vi "SetRF.vi"(0 "reference in":refnum<class "niMmWave_Reciever.lvclass">, 5 "Port":string(combo), 7 "Frequency":dbl format="%#_6pHz", 9 "Gain":dbl format="%#_6fdb", 11 "error in (no error)":errorcluster) -> (4 "reference out":refnum<class "niMmWave_Reciever.lvclass">, 15 "error out":errorcluster)   [LabVIEW 2019, in "niMmWave_Reciever.lvclass"]
doc: "Set RF configuration for port:\nGain and frequency"
uses:
  niMmWave_Reciever.lvclass
  mmWave HW Control/LO sources.ctl
  mmWave HW Control/mmWave HW Control.lvlib
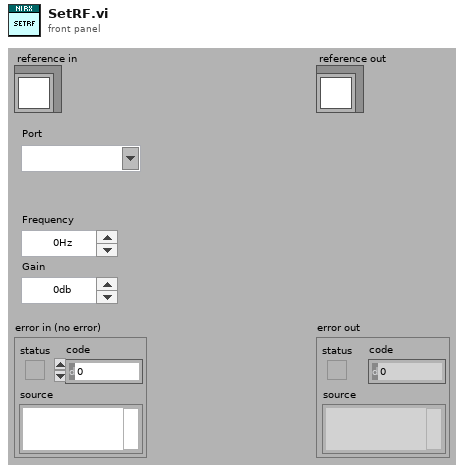
[diagram p1: front panel]
types:
  T1 = typedef "niMmWave_Reciever.lvclass/ObjectAttributesRef.ctl" = refnum<data-value>
  T2 = typedef "niMmWave_Reciever.lvclass/ObjectAttributes.ctl" = cluster{"session":T3[], "HW.RX devices":T17, "RF config":T18, "RX trigger options":T19, "RX samples":i32, "RX Fs":dbl}
  T3 = typedef "Session.ctl" = cluster{"3620 session":refnum<queue>, "tx baseband session":T4, "rx baseband session":T12, "tx gain (dB)":dbl, "rx gain (dB)":dbl, "hardware configuration":T13, "gain ranging":T15[], "pxi trigger bus information":T16}
  T4 = typedef "Tx Baseband Session.ctl" = cluster{"3610 session":T5, "7902 reference":T11}
  T5 = typedef "ni3610_and_ni3630_Driver_Lib.lvlib/Main Settings.ctl" = cluster{"VISA resource name":refnum<visa-resource-name>, "Address Space":T6, "window_offset":u32, "register_addresses":T7, "required_MM_fpga_version":cluster{"signature":u32, "hardware":u32, "current revision":u32, "oldest revision":u32}, "CPLD Oldest Compat Version ":cluster{"hardware":u32, "CPLD firmware":u32}, "MM_FPGA_image_location":string, "is_init":bool, "card_type":T8, "DacLmkConfigFileName":string, "AdcLmkConfigFileName":string, "AdcConfigFileName":string, "DacConfigFileName_RevA":string, "DacConfigFileName_RevB":string, "Mulde hardware revision":u8, "bypass DAC PLL\n":bool, "IQ Card Revision":T9, "board capability":T10}
  T6 = typedef "VISA Register Access Address Space.ctl" = u16
  T7 = typedef "ni3610_and_ni3630_Driver_Lib.lvlib/Register Adresses.ctl" = cluster{"MM based Registers":cluster{"Revision":u32, "OldestCompatRev":u32, "signature":u32, "scratch":u32, "LedControl":u32, "BoardHwRev":u32, "BoardControl":u32, "ThermalStatus":u32, "BasebandStatus":u32, "BasebandControl":u32, "BasebandAuxSetup":u32, "BasebandAuxStatus":u32, "LmkSyncOutSetup":u32, " AdcSyncOutSetup":u32, " InjSyncOutSetup":u32, " PxiTrig0OutSetup":u32, " PxiTrig1OutSetup":u32, " PxiTrig2OutSetup":u32, " PxiTrig3OutSetup":u32, " PxiTrig4OutSetup":u32, " PxiTrig5OutSetup":u32, " PxiTrig6OutSetup":u32, " PxiTrig7OutSetup":u32}, "CPLD based Registers":cluster{"SlaveSignature":u32, "SlaveRevision":u32, "SlaveOldestCompatRev":u32, "SlaveScratch":u32, "SlaveSetup":u32, "SlaveStatus":u32, "IDacReg_offset":u32, "LMKRegGrp0_offset":u32, "QDacReg_offset":u32, "BrdTempSensorVal":u32, "TempSensorPowerDown":u32, "GPIOReg_offset":u32, "IAdcReg_offset":u32, "QAdcReg_offset":u32, "LMKRegGrp1_offset":u32, "QadcTempSensorVal":u32, "IadcTempSensorVal":u32, "RevisionReg":u32, "VcxoReg":u32, "CpldStatusReg":u32, "PowerReg":u32, "VBiasEnReg":u32, "ExtRefOeReg":u32, "QdacCtrlReg":u32, "QdacStatusReg":u32, "IdacCtrlReg":u32, "IdacStatusReg":u32, "QdacJtagIn":u32, "QdacJtagOut":u32, "IdacJtagIn":u32, "IdacJtagOut":u32, "IqDcSetupReg":u32, "QadcStatusReg":u32, "IadcStatusReg":u32, "BrdSetupReg":u32, "IqDcRevisionReg":u32, "PllStatusReg":u32, "EndpointScratchReg":u32, "AdcSyncCfgReg":u32, "IqCardOpampReg":u32}, "CPLD Register Offset":u32, "MM  Register Offset":u32, " PxiTrig0OutSetup":u32}
  T8 = typedef "ni3610_and_ni3630_Driver_Lib.lvlib/Base Card Type.ctl" = enum16{"unspecified", "ADC", "DAC"}
  T9 = typedef "ni3610_and_ni3630_Driver_Lib.lvlib/IQ Card Revision.ctl" = enum16{"RevA", "RevB", "RevC", "RevD"}
  T10 = typedef "ni3610_and_ni3630_Driver_Lib.lvlib/Board Capability.ctl" = cluster{"baseband sync":enum16{"no baseband sync", "baseband sync"}}
  T11 = typedef "Blank FPGA Reference.ctl" = refnum<k20>
  T12 = typedef "Rx Baseband Session.ctl" = cluster{"3630 session":T5, "7902 reference":T11}
  T13 = typedef "Hardware Configuration.ctl" = cluster{"direction":T14, "baseband only":bool}
  T14 = typedef "Direction.ctl" = enum16{"Transceiver", "Receiver", "Transmitter"}
  T15 = typedef "Gain Ranging.ctl" = cluster{"gain ranging active scope":string, "gain ranging stream session":refnum<k20>}
  T16 = typedef "PXI Trigger Bus Info.ctl" = cluster{"chassis resource name":refnum<visa-resource-name>, "7902R (TX)":i16, "3610 (TX)":i16, "3620 (IF)":i16, "3630 (RX)":i16, "7902R (RX)":i16}
  T17 = typedef "mmWave HW Control.lvlib/HW RX resources cluster.ctl" = cluster{"HW.IF":tag, "HW.ADC":refnum<visa-resource-name>, "HW.RX FPGA":tag}
  T18 = typedef "mmWave HW Control.lvlib/HW RX RF config cluster.ctl" = cluster{"Gain":dbl, "Frequency":dbl, "mmWave adapter":string}
  T19 = typedef "TX trigger config.ctl" = cluster{"delay":dbl, "trig source":T20, "PXI src":i32, "export":T21, "PXI dest":i32}
  T20 = typedef "FPGA Utility.lvlib/FPGA driver trigger source.ctl" = enum16{"Use Tclk", "PXI_Trig", "Aurora RX trig"}
  T21 = typedef "FPGA Utility.lvlib/FPGA driver trigger destination.ctl" = enum16{"None", "Source trig", "Synced trig", "Delayed sync"}
  T22 = typedef "mmWave HW Control.lvlib/LO sources.ctl" = cluster{"RX/LO1 src":string, "TX/LO1 src":string, "LO2 src":string}
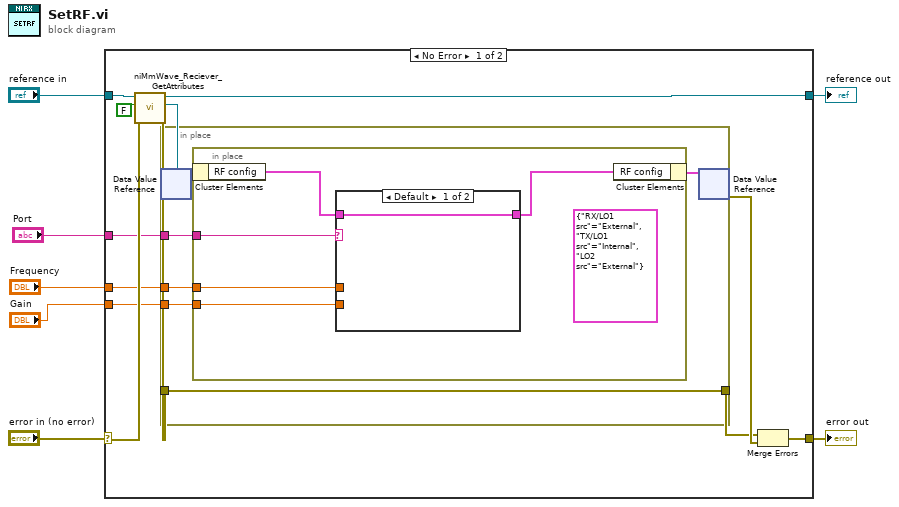
[diagram p0: block diagram]
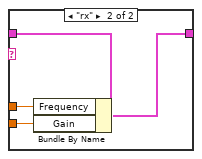
[diagram p2: hidden frame]
diagram:
  n1 = case shown="No Error" "error in (no error)" {
    selector: "error in (no error)" -> [w14 w37]
    tunnel: [w19 w37] -> w6
    tunnel: [w12 w36] -> w4
    tunnel: "reference in" -> [w16 w36]
    tunnel: "Port" -> [w10 _]
    tunnel: "Frequency" -> [w9 _]
    tunnel: "Gain" -> [w8 _]
    frame No Error {
      n2 = call "niMmWave_Reciever_GetAttributes.vi"("error in (no error)"=w14, "return data? (T)"=FALSE, "reference in"=w16) -> ("error out"=w13:errorcluster, "attributes ref"=w11:T1, "reference out"=w12:refnum<class "niMmWave_Reciever.lvclass">)  [unwired: 5 in, 1 out]
      n3 = in-place {
        in-place-border: w13 -> [w23]
        in-place-border: [w23] -> w17
        in-place-border: w10 -> [w22]
        in-place-border: w9 -> [w21]
        in-place-border: w8 -> [w20]
        n4 = in-place-dvr #1(w11) -> (w24:T2)  [unwired: 1 out]
        n5 = in-place {
          in-place-border: w22 -> [w28]
          in-place-border: w21 -> [w27]
          in-place-border: w20 -> [w26]
          (unwired) T22 {"RX/LO1 src"="External", "TX/LO1 src"="Internal", "LO2 src"="External"} ("LO sources")
          n6 = in-place-cluster #2(w24) -> ("RF config"=w29:T18)
          n7 = case shown="Default" w28 {
            tunnel: [w31 w34] -> w30
            tunnel: w29 -> [w31 w35]
            tunnel: w27 -> [_ w33]
            tunnel: w26 -> [_ w32]
            frame Default {
            }
            frame "rx" {
              n8 = Bundle By Name(cluster=w35, "Frequency"=w33, "Gain"=w32) -> (w34:T18)
            }
          }
          n9 = in-place-cluster #2("RF config"=w30) -> (w25:T2)
        }
        n10 = in-place-dvr #1(w25) -> (w18:errorcluster)  [unwired: 1 out]
      }
      n11 = Merge Errors(w17, w18) -> (w19:errorcluster)
    }
    frame Error {
    }
  }
  "error out" <- w6
  "reference out" <- w4
